vi "save_summary_data.vi"(8 "LAST VALVE":i32, 9 "#of reactors":i32, 10 "REACTORS":T1(array[cluster]), 11 "summary file":path=path "C:/Documents and Settings/Administrator/Desktop/BIOREACTOR 2/experiments/20140703tests.csv") -> ()   [LabVIEW 2013]
uses:
  <vilib>/Utility/file.llb/Write To Spreadsheet File (DBL).vi
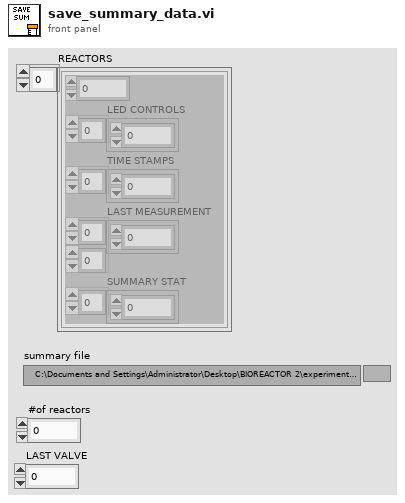
[diagram p1: front panel]
types:
  T1 = cluster{i32, "LED CONTROLS":dbl[], "TIME STAMPS":dbl[], "LAST MEASUREMENT":dbl[][], "SUMMARY STAT":dbl[]}[]
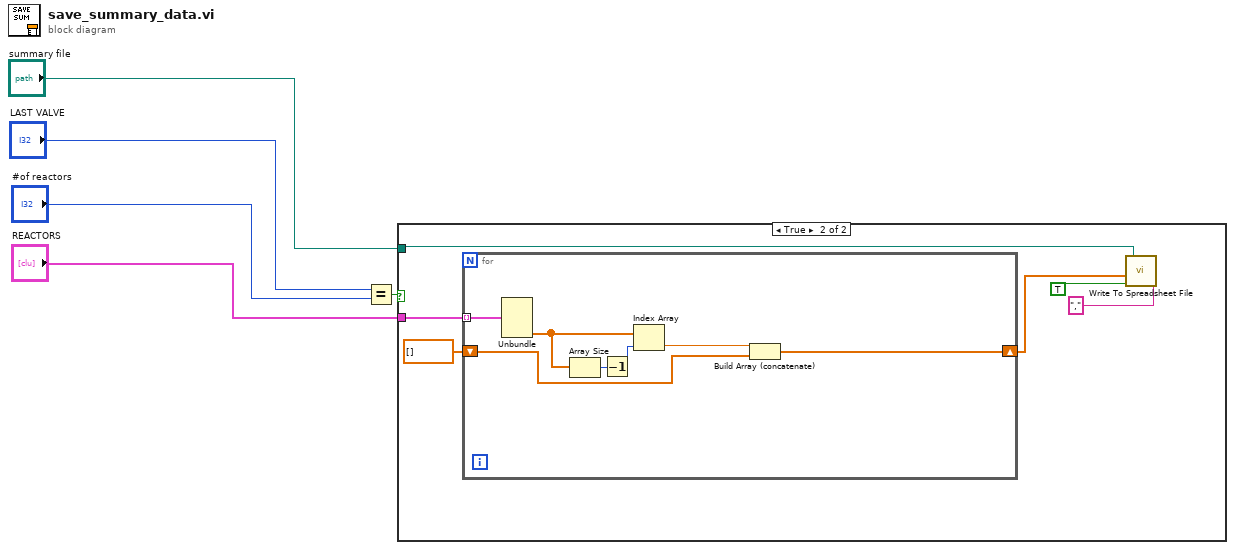
[diagram p0: block diagram]
diagram:
  n1 = Equal?(x="LAST VALVE", y="#of reactors") -> (x = y?=w5:bool)
  n2 = case shown="True" w5 {
    tunnel: "summary file" -> [_ w10]
    tunnel: "REACTORS" -> [_ w8]
    frame False {
    }
    frame True {
      n3 = for {
        tunnel: w8 -> [w18] mode=indexing
        shift-right: [w13] -> w7
        shift-left: dbl[] [] -> [w12]
        n4 = Unbundle(w18) -> ("SUMMARY STAT"=w17:dbl[])  [unwired: 4 out]
        n5 = Array Size(array=w17) -> (size(s)=w16:i32)
        n6 = Decrement(x=w16) -> (x-1=w15:i32)
        n7 = Index Array(array=w17, index=w15) -> (element=w14:dbl)
        n8 = Build Array (concatenate)(w14, w12) -> (w13:dbl[])
      }
      n9 = call-poly <vilib>:"Write To Spreadsheet File.vi"("delimiter (\\t)"="," ("delimiter (\\t)"), "append to file? (new file:F)"=TRUE, "1D data"=w7, "file path (dialog if empty)"=w10) -> ()  [unwired: 4 in, 1 out]
    }
  }
